vi "VisionDashRead_FrontRight.vi"() -> (0 "FR Ang Deg":dbl, 1 "FR Y Ft":dbl, 2 "FR X Ft":dbl, 3 "FR Error":bool, 4 "FR Time Sec":dbl, 5 "FR Conn":bool, 6 "FR Last Sec Cnt":i64, 7 "FR HasTarg":bool, 8 "FR Count":i64, 11 "FR NewData":bool)   [LabVIEW 2023]
doc: "Vision Network\n\nInput\n --Error in \n\nOutput\n --Error out"
uses:
  <vilib>/Rock Robotics/Network Tables/NT Read Integer.vi
  <vilib>/Rock Robotics/Network Tables/NT Read Boolean.vi
  <vilib>/Rock Robotics/Network Tables/NT Read Number.vi
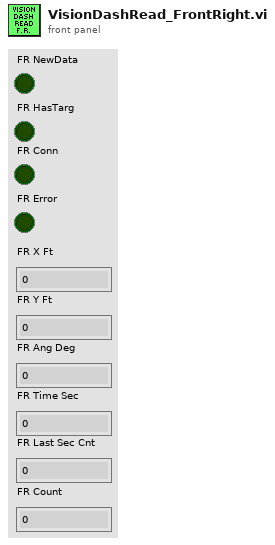
[diagram p1: front panel]
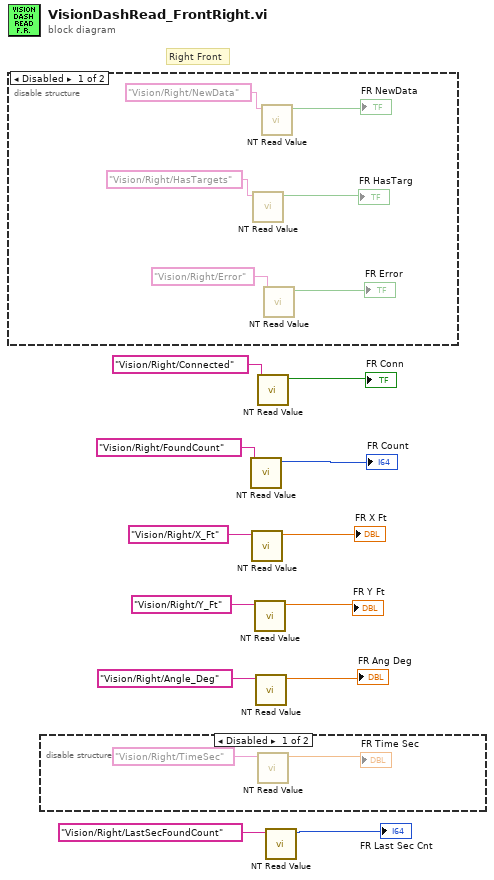
[diagram p0: block diagram]
diagram:
  # "Right Front"
  n1 = disable-structure shown="Disabled" {
    frame Disabled {
      n2 = call-poly <vilib>:"NT Read Value.vi"("name"="Vision/Right/HasTargets") -> ("value"=→"FR HasTarg":bool)  [unwired: 8 in, 2 out]
      n3 = call-poly <vilib>:"NT Read Value.vi"("name"="Vision/Right/NewData") -> ("value"=→"FR NewData":bool)  [unwired: 8 in, 2 out]
      n4 = call-poly <vilib>:"NT Read Value.vi"("name"="Vision/Right/Error") -> ("value"=→"FR Error":bool)  [unwired: 8 in, 2 out]
    }
    frame Enabled {
    }
  }
  n5 = disable-structure shown="Disabled" {
    frame Disabled {
      n6 = call-poly <vilib>:"NT Read Value.vi"("name"="Vision/Right/TimeSec") -> ("value"=→"FR Time Sec":dbl)  [unwired: 8 in, 2 out]
    }
    frame Enabled {
    }
  }
  n7 = call-poly <vilib>:"NT Read Value.vi"("name"="Vision/Right/FoundCount") -> ("value"=→"FR Count":i64)  [unwired: 8 in, 2 out]
  n8 = call-poly <vilib>:"NT Read Value.vi"("name"="Vision/Right/X_Ft") -> ("value"=→"FR X Ft":dbl)  [unwired: 8 in, 2 out]
  n9 = call-poly <vilib>:"NT Read Value.vi"("name"="Vision/Right/Y_Ft") -> ("value"=→"FR Y Ft":dbl)  [unwired: 8 in, 2 out]
  n10 = call-poly <vilib>:"NT Read Value.vi"("name"="Vision/Right/Angle_Deg") -> ("value"=→"FR Ang Deg":dbl)  [unwired: 8 in, 2 out]
  n11 = call-poly <vilib>:"NT Read Value.vi"("name"="Vision/Right/Connected") -> ("value"=→"FR Conn":bool)  [unwired: 8 in, 2 out]
  n12 = call-poly <vilib>:"NT Read Value.vi"("name"="Vision/Right/LastSecFoundCount") -> ("value"=→"FR Last Sec Cnt":i64)  [unwired: 8 in, 2 out]
